vi "MAT Save Matrix.vi"(0 "Ref Num":refnum<file>, 1 "DBL":dbl[][](array[numeric]) format="%.2f", 2 "SGL":sgl[][](array[numeric]) format="%.2f", 3 "I32":i32[][](array[numeric]), 4 "I16":i16[][](array[numeric]), 5 "error in":errorcluster, 6 "Matrix Name":string, 7 "U16":u16[][](array[numeric]), 8 "offset in (-1: current position)":i64=-1, 9 "U8":u8[][](array[numeric]), 10 "STR":string[](array[string]), 11 "CDB":cdb[][](array[numeric]) format="%.2f", 13 "CSG":csg[][](array[numeric]) format="%.2f") -> (14 "Dup Ref Num":refnum<file>, 19 "error out":errorcluster)   [LabVIEW 2013]
doc: "\"Save to MAT\" saves a 2D array of numbers or a 1D array of strings to MATLAB file. It works only with LabVIEW for Windows. All data types, described in MATLAB/External Interface Guide/Appendix A, are supported, except Sparse Matrices.\n\nAll data inputs should be 2D arrays, except String input which should be a 1D array. Only one data input may contain a non-empty array, otherwise error will be generated (error code -1).\n\nSAVML.LLB is a freeware written by Serge Liberman <liber@us1.channel1.com>."
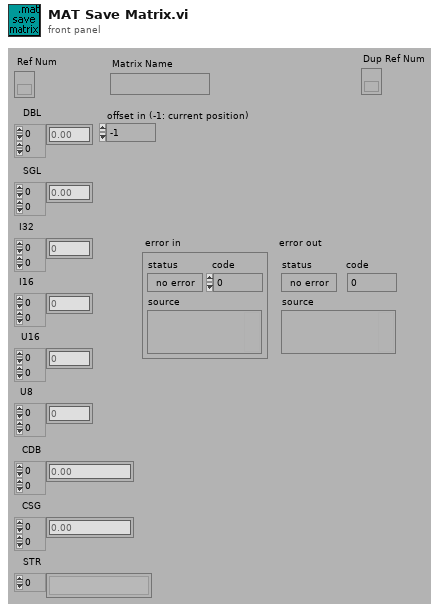
[diagram p1: front panel]
types:
  T1 = enum16{"big-endian, network order", "native, host order", "little-endian"}
  T2 = typedef "MAT Type Representation.ctl" = enum16{"DBL", "SGL", "I32", "I16", "U16", "U8", "CDB", "CSG", "STR"}
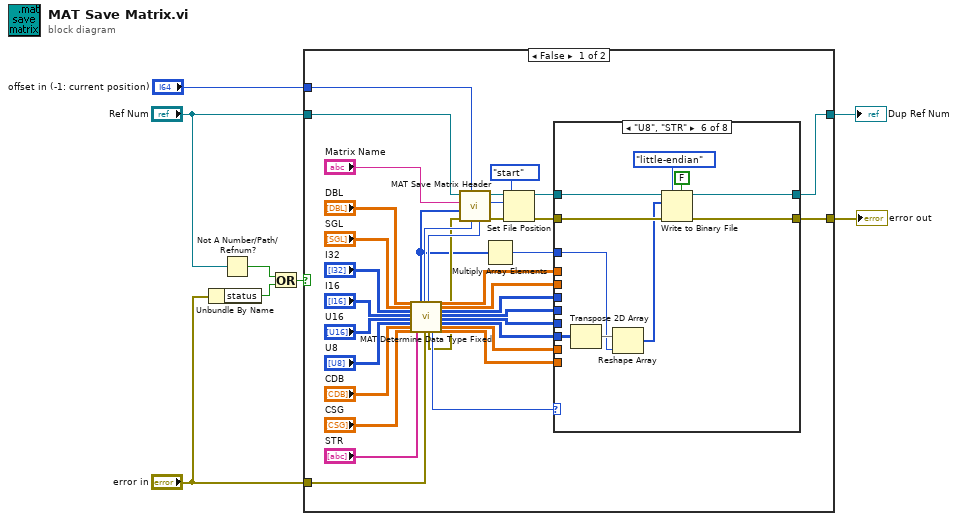
[diagram p0: block diagram]
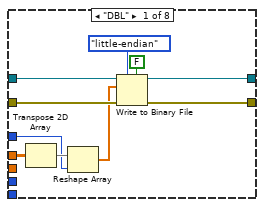
[diagram p2: hidden frame]
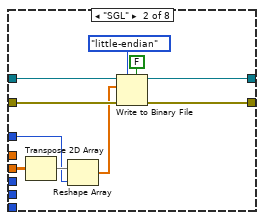
[diagram p3: hidden frame]
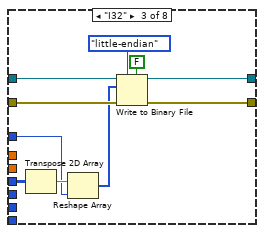
[diagram p4: hidden frame]
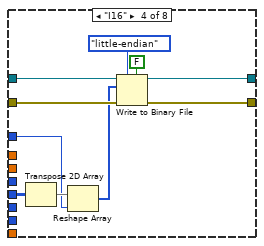
[diagram p5: hidden frame]
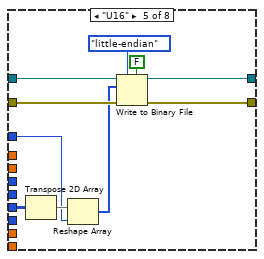
[diagram p6: hidden frame]
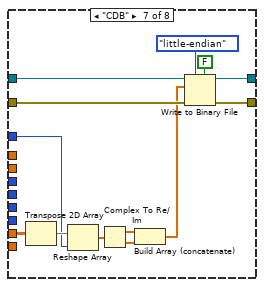
[diagram p7: hidden frame]
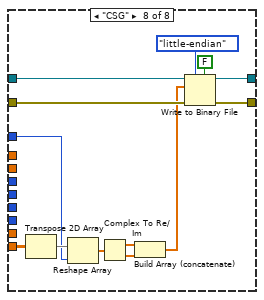
[diagram p8: hidden frame]
diagram:
  n1 = Unbundle By Name("error in") -> ("status"=w5:bool)
  n2 = Not A Number/Path/Refnum?(number/path/refnum="Ref Num") -> (NaN/Path/Refnum?=w3:bool)
  n3 = Or(x=w3, y=w5) -> (x .or. y?=w2:bool)
  n4 = case shown="False" w2 {
    tunnel: [w10 w131] -> w8
    tunnel: "Ref Num" -> [w43 w131]
    tunnel: "error in" -> [w20 w130]
    tunnel: [w42 w130] -> w6
    tunnel: "offset in (-1: current position)" -> [w9 _]
    frame False {
      n5 = call "MAT Determine Data Type Fixed.vi"("DBL"="DBL", "SGL"="SGL", "I32"="I32", "I16"="I16", "U16"="U16", "U8"="U8", "CDB"="CDB", "CSG"="CSG", "STR"="STR", "error in (no error)"=w20) -> ("Matrix Size"=w18:i32[], "Rep. Code"=w22:u32, "Real/Complex (0-Real)"=w23:u32, "error out"=w19:errorcluster, "Representation"=w21:T2, "DBL copy"=w31:dbl[][], "SGL copy"=w30:sgl[][], "I32 copy"=w29:i32[][], "I16 copy"=w28:i16[][], "U16 copy"=w27:u16[][], "U8 copy"=w26:u8[][], "CDB copy"=w25:cdb[][], "CSG copy"=w24:csg[][])  [unwired: 5 in]
      n6 = call "MAT Save Matrix Header.vi"("Real/Complex (0-Real)"=w23, "Rep. Code"=w22, "offset in (-1: current position)"=w9, "error in (no error)"=w19, "Matrix Size"=w18, "Matrix Name"="Matrix Name", "Ref Num"=w43) -> ("error out"=w16:errorcluster, "offset out"=w12:i64, "Dup Ref Num"=w14:refnum<file>)  [unwired: 2 in]
      n7 = Multiply Array Elements(1:w18) -> (0:w17:i32)
      n8 = Set File Position(offset (in bytes) (0)=w12, refnum=w14, from (0:start)=enum16{"start", "end", "current"}."start", error in=w16) -> (refnum out=w13:refnum<file>, error out=w15:errorcluster)
      n9 = case shown="\"U8\", \"STR\"" w21 {
        tunnel: w13 -> [w49 w60 w70 w80 w90 w100 w113 w126]
        tunnel: w31 -> [w53 _ _ _ _ _ _ _]
        tunnel: w30 -> [_ w54 _ _ _ _ _ _]
        tunnel: w29 -> [_ _ w64 _ _ _ _ _]
        tunnel: w28 -> [_ _ _ w74 _ _ _ _]
        tunnel: w27 -> [_ _ _ _ w84 _ _ _]
        tunnel: w26 -> [_ _ _ _ _ w94 _ _]
        tunnel: w25 -> [_ _ _ _ _ _ w108 _]
        tunnel: w24 -> [_ _ _ _ _ _ _ w117]
        tunnel: [w44 w55 w65 w75 w85 w95 w109 w122] -> w10
        tunnel: w15 -> [w50 w61 w71 w81 w91 w101 w114 w127]
        tunnel: [w45 w56 w66 w76 w86 w96 w110 w123] -> w42
        tunnel: w17 -> [w51 w62 w72 w82 w92 w102 w115 w128]
        frame "DBL" {
          n10 = Transpose 2D Array(2D array=w53) -> (transposed array=w52:dbl[][])
          n11 = Reshape Array(w52, w51) -> (w48:dbl[])
          n12 = Write to Binary File(file (use dialog)=w49, data=w48, error in=w50, 5:FALSE ("prepend array or string size? (T)"), 9:T1."little-endian" ("byte order (0:big-endian, network order)")) -> (refnum out=w44:refnum<file>, error out=w45:errorcluster)  [unwired: 1 in, 1 out]
        }
        frame "SGL" {
          n13 = Transpose 2D Array(2D array=w54) -> (transposed array=w63:sgl[][])
          n14 = Reshape Array(w63, w62) -> (w59:sgl[])
          n15 = Write to Binary File(file (use dialog)=w60, data=w59, error in=w61, 5:FALSE ("prepend array or string size? (T)"), 9:T1."little-endian" ("byte order (0:big-endian, network order)")) -> (refnum out=w55:refnum<file>, error out=w56:errorcluster)  [unwired: 1 in, 1 out]
        }
        frame "I32" {
          n16 = Transpose 2D Array(2D array=w64) -> (transposed array=w73:i32[][])
          n17 = Reshape Array(w73, w72) -> (w69:i32[])
          n18 = Write to Binary File(file (use dialog)=w70, data=w69, error in=w71, 5:FALSE ("prepend array or string size? (T)"), 9:T1."little-endian" ("byte order (0:big-endian, network order)")) -> (refnum out=w65:refnum<file>, error out=w66:errorcluster)  [unwired: 1 in, 1 out]
        }
        frame "I16" {
          n19 = Transpose 2D Array(2D array=w74) -> (transposed array=w83:i16[][])
          n20 = Reshape Array(w83, w82) -> (w79:i16[])
          n21 = Write to Binary File(file (use dialog)=w80, data=w79, error in=w81, 5:FALSE ("prepend array or string size? (T)"), 9:T1."little-endian" ("byte order (0:big-endian, network order)")) -> (refnum out=w75:refnum<file>, error out=w76:errorcluster)  [unwired: 1 in, 1 out]
        }
        frame "U16" {
          n22 = Transpose 2D Array(2D array=w84) -> (transposed array=w93:u16[][])
          n23 = Reshape Array(w93, w92) -> (w89:u16[])
          n24 = Write to Binary File(file (use dialog)=w90, data=w89, error in=w91, 5:FALSE ("prepend array or string size? (T)"), 9:T1."little-endian" ("byte order (0:big-endian, network order)")) -> (refnum out=w85:refnum<file>, error out=w86:errorcluster)  [unwired: 1 in, 1 out]
        }
        frame "U8", "STR" {
          n25 = Transpose 2D Array(2D array=w94) -> (transposed array=w103:u8[][])
          n26 = Reshape Array(w103, w102) -> (w99:u8[])
          n27 = Write to Binary File(file (use dialog)=w100, data=w99, error in=w101, 5:FALSE ("prepend array or string size? (T)"), 9:T1."little-endian" ("byte order (0:big-endian, network order)")) -> (refnum out=w95:refnum<file>, error out=w96:errorcluster)  [unwired: 1 in, 1 out]
        }
        frame "CDB" {
          n28 = Transpose 2D Array(2D array=w108) -> (transposed array=w116:cdb[][])
          n29 = Reshape Array(w116, w115) -> (w107:cdb[])
          n30 = Complex To Re/Im(x + iy=w107) -> (x=w106:dbl[], y=w105:dbl[])
          n31 = Build Array (concatenate)(w106, w105) -> (w104:dbl[])
          n32 = Write to Binary File(file (use dialog)=w113, data=w104, error in=w114, 5:FALSE ("prepend array or string size? (T)"), 9:T1."little-endian" ("byte order (0:big-endian, network order)")) -> (refnum out=w109:refnum<file>, error out=w110:errorcluster)  [unwired: 1 in, 1 out]
        }
        frame "CSG" {
          n33 = Transpose 2D Array(2D array=w117) -> (transposed array=w129:csg[][])
          n34 = Reshape Array(w129, w128) -> (w121:csg[])
          n35 = Complex To Re/Im(x + iy=w121) -> (x=w120:sgl[], y=w119:sgl[])
          n36 = Build Array (concatenate)(w120, w119) -> (w118:sgl[])
          n37 = Write to Binary File(file (use dialog)=w126, data=w118, error in=w127, 5:FALSE ("prepend array or string size? (T)"), 9:T1."little-endian" ("byte order (0:big-endian, network order)")) -> (refnum out=w122:refnum<file>, error out=w123:errorcluster)  [unwired: 1 in, 1 out]
        }
      }
    }
    frame True {
    }
  }
  "error out" <- w6
  "Dup Ref Num" <- w8
